vi "Config Spectrometer.vi"(4 "Laser Led Select (Laser)":enum16{"Laser", "Led"}(ring), 6 "Ref Lvl Auto":bool, 7 "Valor de Span (nm)":dbl=100.0, 8 "error in (no error)":errorcluster, 9 "Centro do Pico do espectro (nm)":dbl=1550.0, 10 "Resolution":enum16{"Normal", "High"}(ring), 11 "VISA Refnum in":refnum<visa-resource-name>="GPIB0::9::INSTR") -> (0 "error out":errorcluster, 3 "VISA Refnum out":refnum<visa-resource-name>)   [LabVIEW 2021]
uses:
  f45516d5-78c5-4aba-88ba-dcf34f3dc23c.vi
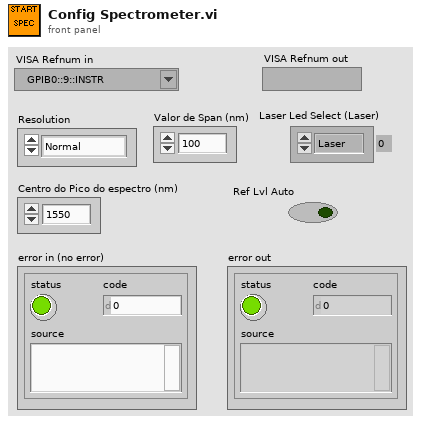
[diagram p1: front panel]
types:
  T1 = enum16{"um", "nm", "nm/DIV", "mm", "THz", "GHz", "THz/DIV", "GHz/DIV"}
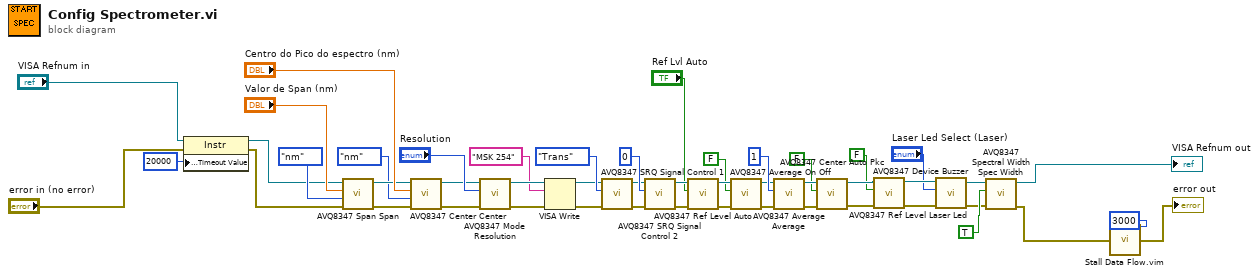
[diagram p0: block diagram]
diagram:
  n1 = property class="Instr"(reference="VISA Refnum in", error in="error in (no error)", "General Settings:Timeout Value"=u32 20000) -> (reference out=w14:refnum<visa-resource-name>, error out=w13:errorcluster)
  n2 = call "AVQ8347 Span Span.vi"("Error In"=w13, "Span Unit (nm)"=T1."nm", "Span Value (700)"="Valor de Span (nm)", "VISA Session"=w14) -> ("Error Out"=w39:errorcluster, "Copy VISA Session"=w40:refnum<visa-resource-name>)  [unwired: 5 in, 1 out]
  n3 = call "AVQ8347 Center Center.vi"("Error In"=w39, "Center Point Unit (nm)"=enum16{"um", "nm", "THz", "GHz"}."nm", "Center Point Value (700)"="Centro do Pico do espectro (nm)", "VISA Session"=w40) -> ("Error Out"=w37:errorcluster, "Copy VISA Session"=w36:refnum<visa-resource-name>)  [unwired: 5 in, 1 out]
  n4 = call "AVQ8347 Mode Resolution.vi"("Error In"=w37, "Mode Select (Normal)"="Resolution", "VISA Session"=w36) -> ("Error Out"=w34:errorcluster, "Copy VISA Session"=w35:refnum<visa-resource-name>)  [unwired: 6 in, 1 out]
  n5 = VISA Write(VISA resource name=w35, write buffer="MSK 254", error in (no error)=w34) -> (VISA resource name out=w21:refnum<visa-resource-name>, error out=w20:errorcluster)  [unwired: 1 out]
  n6 = call "AVQ8347 SRQ Signal Control 1.vi"("Error In"=w20, "SRQ Trans Sel (No Trans)"=enum16{"No Trans", "Trans"}."Trans", "VISA Session"=w21) -> ("Error Out"=w18:errorcluster, "Copy VISA Session"=w19:refnum<visa-resource-name>)  [unwired: 6 in, 1 out]
  n7 = call "AVQ8347 SRQ Signal Control 2.vi"("Error In"=w18, "SRQ Trans Sel (No Trans)"=u16 0 ("Average Value (1)"), "VISA Session"=w19) -> ("Error Out"=w46:errorcluster, "Copy VISA Session"=w45:refnum<visa-resource-name>)  [unwired: 6 in, 1 out]
  n8 = call "AVQ8347 Ref Level Auto.vi"("Error In"=w46, "Mode selection (OFF)"="Ref Lvl Auto", "VISA Session"=w45) -> ("Error Out"=w30:errorcluster, "Copy VISA Session"=w31:refnum<visa-resource-name>)  [unwired: 6 in, 1 out]
  n9 = call "AVQ8347 Average On Off.vi"("Error In"=w30, "Processing Select (OFF)"=FALSE, "VISA Session"=w31) -> ("Error Out"=w29:errorcluster, "Copy VISA Session"=w28:refnum<visa-resource-name>)  [unwired: 6 in, 1 out]
  n10 = call "AVQ8347 Average Average.vi"("Error In"=w29, "Average Value (1)"=u16 1, "VISA Session"=w28) -> ("Error Out"=w25:errorcluster, "Copy VISA Session"=w26:refnum<visa-resource-name>)  [unwired: 6 in, 1 out]
  n11 = call "AVQ8347 Center Auto Pkc.vi"("Error In"=w25, "APC Function selection (OFF)"=FALSE, "VISA Session"=w26) -> ("Error Out"=w12:errorcluster, "Copy VISA Session"=w11:refnum<visa-resource-name>)  [unwired: 6 in, 1 out]
  n12 = call "AVQ8347 Device Buzzer.vi"("Error In"=w12, "Buzzer Control (OFF)"=FALSE, "VISA Session"=w11) -> ("Error Out"=w5:errorcluster, "Copy VISA Session"=w8:refnum<visa-resource-name>)  [unwired: 6 in, 1 out]
  n13 = call "AVQ8347 Ref Level Laser Led.vi"("Error In"=w5, "Laser Led Select (Laser)"="Laser Led Select (Laser)", "VISA Session"=w8) -> ("Error Out"=w4:errorcluster, "Copy VISA Session"=w2:refnum<visa-resource-name>)  [unwired: 6 in, 1 out]
  n14 = call "AVQ8347 Spectral Width Spec Width.vi"("Error In"=w4, "Half Width (OFF)"=TRUE, "VISA Session"=w2) -> ("Error Out"=w3:errorcluster, "Copy VISA Session"=→"VISA Refnum out":refnum<visa-resource-name>)  [unwired: 6 in, 1 out]
  n15 = call "Stall Data Flow.vim"("value in"=w3, "milliseconds to wait"=u32 3000) -> ("value out"=→"error out":errorcluster)  [unwired: 1 out]
